vi "Final LCD Input Enum.vi"() -> ()   [LabVIEW 2017]
uses:
  controls/StatesEnum.ctl
panel:
  in  "String Input":string
  out "error out":errorcluster
  in  "error in (no error)":errorcluster
  in  "state input":T1=enum."Shut"
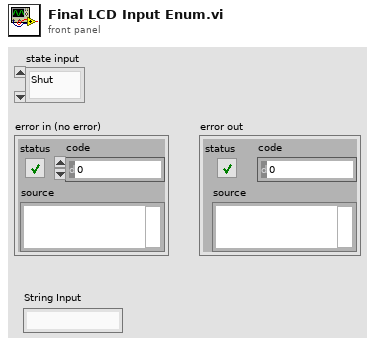
[diagram p1: front panel]
types:
  T1 = typedef "StatesEnum.ctl" = enum16{"Init", "Center Cliff\n", "Pause", "Drive", "L.Cliff", "R.Cliff", "Shut"}
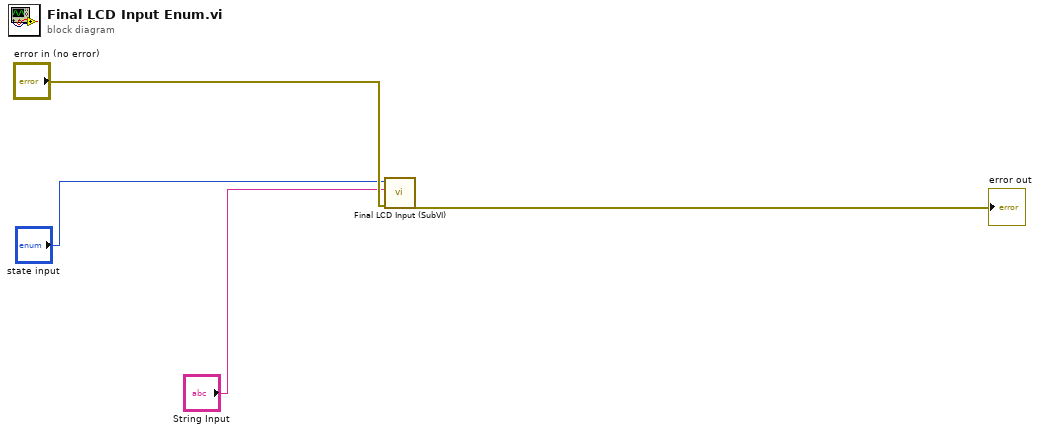
[diagram p0: block diagram]
diagram:
  n1 = call "Final LCD Input (SubVI).vi"("error in (no error)"="error in (no error)", "String Input"="String Input", "state input"="state input") -> ("error out"=→"error out":errorcluster)  [unwired: 8 in]
